vi "首页显示设置.vi"() -> ()   [LabVIEW 2016]
uses:
  <vilib>/Utility/config.llb/NI_LVConfig.lvlib
panel:
  in  "首页显示信息设置":T1
  in  "关闭":bool
  # "首页显示信息设置"
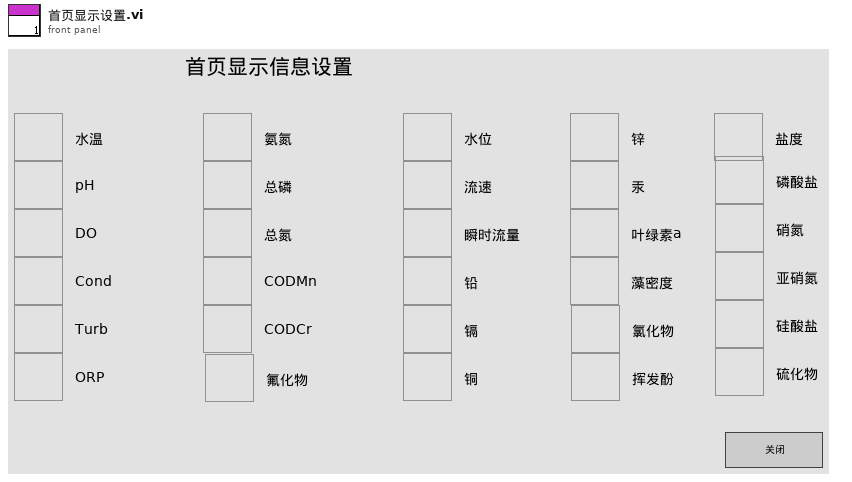
[diagram p1: front panel]
types:
  T1 = cluster{"水温":bool, "pH":bool, "DO":bool, "Cond":bool, "Turb":bool, "氨氮":bool, "总磷":bool, "总氮":bool, "CODMn":bool, "CODCr":bool, "水位":bool, "流速":bool, "瞬时流量":bool, "Turb 2":bool, "氟化物":bool, "铅":bool, "镉":bool, "铜":bool, "锌":bool, "汞":bool, "叶绿素a":bool, "藻密度":bool, "氯化物":bool, "挥发酚":bool, "盐度":bool, "磷酸盐":bool, "硝氮":bool, "亚硝氮":bool, "硅酸盐":bool, "硫化物":bool}
  T2 = cluster{"水温":bool, "pH":bool, "DO":bool, "Cond":bool, "Turb":bool, "氨氮":bool, "总磷":bool, "总氮":bool, "CODMn":bool, "CODCr":bool, "水位":bool, "流速":bool, "瞬时流量":bool, "ORP":bool, "氟化物":bool, "铅":bool, "镉":bool, "铜":bool, "锌":bool, "汞":bool, "叶绿素a":bool, "藻密度":bool, "氯化物":bool, "挥发酚":bool, "盐度":bool, "磷酸盐":bool, "硝氮":bool, "亚硝氮":bool, "硅酸盐":bool, "硫化物":bool}
  T3 = typedef "NI_LVConfig.lvlib/Config Data RefNum.ctl" = refnum<k1>
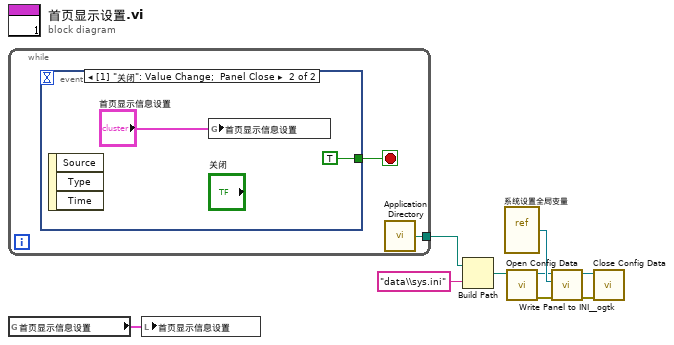
[diagram p0: block diagram]
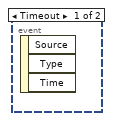
[diagram p2: hidden frame]
diagram:
  n1 = while {
    tunnel: [w10] -> w2
    stop <- w11 stop-if-true
    n2 = event shown="[1] \"关闭\": Value Change;  Panel Close" {
      selector: _ -> [_ _]
      dyn-events: _ -> [_ _]
      timeout: _ -> [_ _]
      tunnel: [_ TRUE] -> w11
      event Timeout {
        n3 = event-data() -> ()  [unwired: 1 in, 3 out]
      }
      event "关闭": Value Change; Panel Close {
        n4 = event-data() -> ()  [unwired: 1 in, 3 out]
        n5 = global write "系统设置全局变量.vi" "首页显示信息设置"("首页显示信息设置") -> ()
      }
    }
    n6 = call <vilib>:"Application Directory.vi"() -> ("Application Directory"=w10:path)
  }
  n7 = global read "系统设置全局变量.vi" "首页显示信息设置"() -> (w1:T2)
  n8 = local write "首页显示信息设置"(w1) -> ()
  n9 = Build Path(base path=w2, name or relative path="data\\sys.ini" ("名称或相对路径")) -> (appended path=w4:path)
  n10 = vi-ref "系统设置全局变量.vi"() -> (w6:refnum<vi>)
  n11 = call <vilib>:"Open Config Data.vi"("configuration file path"=w4) -> ("error out"=w8:errorcluster, "refnum"=w5:T3)  [unwired: 8 in, 1 out]
  n12 = call <userlib>:"Write Panel to INI__ogtk.vi"("error in (no error)"=w8, "VI ref"=w6, "refnum"=w5) -> ("error out"=w9:errorcluster, "refnum out"=w7:T3)  [unwired: 7 in]
  n13 = call <vilib>:"Close Config Data.vi"("error in (no error)"=w9, "refnum"=w7) -> ()  [unwired: 8 in, 2 out]
